vi "RunTimeMenu Wrapper.vi"(8 "error in":errorcluster, 11 "Node Ptr":u64 format="%.0x") -> (0 "error out":errorcluster)   [LabVIEW 2020, in "AIM MIL-STD-1553 System Explorer.lvlib"]
uses:
  AIM MIL-STD-1553 System Explorer.lvlib
  Includes/AIM MIL-STD-1553 System Explorer.lvlibp/System Explorer/Interfaces/System Explorer Dispatcher/System Explorer Dispatcher.lvclass
  Includes/AIM MIL-STD-1553 System Explorer.lvlibp/System Explorer/Implementation/System Explorer Dispatcher/System Explorer Dispatcher.lvclass
  C:/dev/git/niveristand-aim-milStd1553-custom-device/Includes/AIM MIL-STD-1553 System Explorer.lvlibp/System Explorer/Interfaces/System Explorer Dispatcher/System Explorer Dispatcher.lvclass
panel:
  in  "tag":string
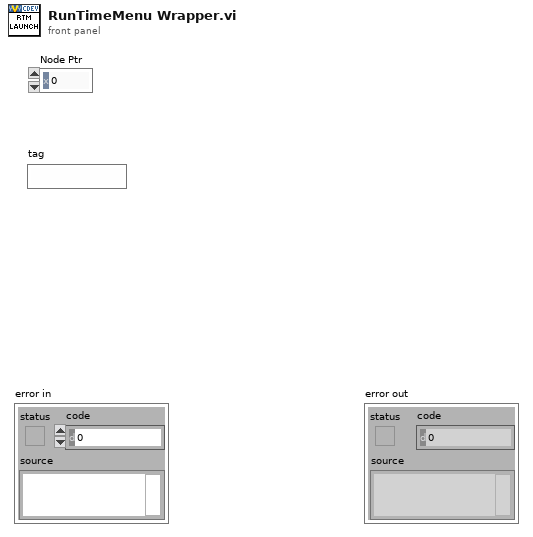
[diagram p1: front panel]
types:
  T1 = typedef "Custom Device API.lvlib/Custom Device Item Ref.ctl" = u64
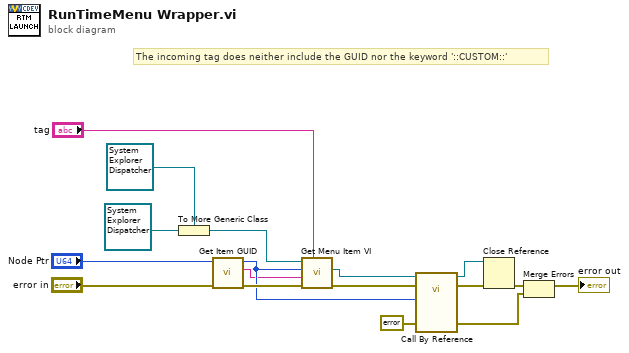
[diagram p0: block diagram]
diagram:
  # "The incoming tag does neither include the GUID nor the keyword '::CUSTOM::'"
  n1 = To More Generic Class(target class=refnum<class "System Explorer Dispatcher.lvclass"> refnum ("AIM MIL-STD-1553 System Explorer.lvlibp:Interfaces.lvlib:System Explorer Dispatcher.lvclass"), reference=refnum<class "System Explorer Dispatcher.lvclass"> refnum ("AIM MIL-STD-1553 System Explorer.lvlibp:Implementation.lvlib:System Explorer Dispatcher.lvclass")) -> (generic class reference=w17:refnum<class "System Explorer Dispatcher.lvclass">)
  n2 = call "Get Item GUID.vi"("error in (no error)"="error in", "item in"="Node Ptr") -> ("error out"=w4:errorcluster, "guid"=w2:string, "item out"=w3:T1)  [unwired: 7 in]
  n3 = call-dynamic "Get Menu Item VI.vi"("Menu Item"="tag", "error in (no error)"=w4, "GUID"=w2, "Item Ref"=w3, "System Explorer Dispatcher in"=w17) -> ("error out"=w15:errorcluster, "menu item reference"=w16:refnum<vi>)  [unwired: 4 in, 1 out]
  n4 = call-by-ref "?"(reference=w16, error in=w15, 8:"error in (no error)"=errorcluster {"status"=FALSE, "code"=0, "source"=""} ("error in"), "Node Ptr"=w3) -> (reference out=w12:refnum<vi>, error out=w13:errorcluster, 0:"error out"=w8:errorcluster)  [unwired: 9 in]
  n5 = Close Reference(reference=w12, error in (no error)=w13) -> (error out=w11:errorcluster)
  n6 = Merge Errors(w11, w8) -> (→"error out":errorcluster)
